vi "Merge Load Steps.vi"(9 "Load Steps  In 2":T1[](array[typedef]), 10 "Load Steps In":T1[](array[typedef])) -> (2 "Load Steps Out":T1[](array[typedef]))   [LabVIEW 2009]
uses:
  Load Step.ctl
  Widget/Target.ctl
  Data Access Objects/Metadata/LBCB Number.ctl
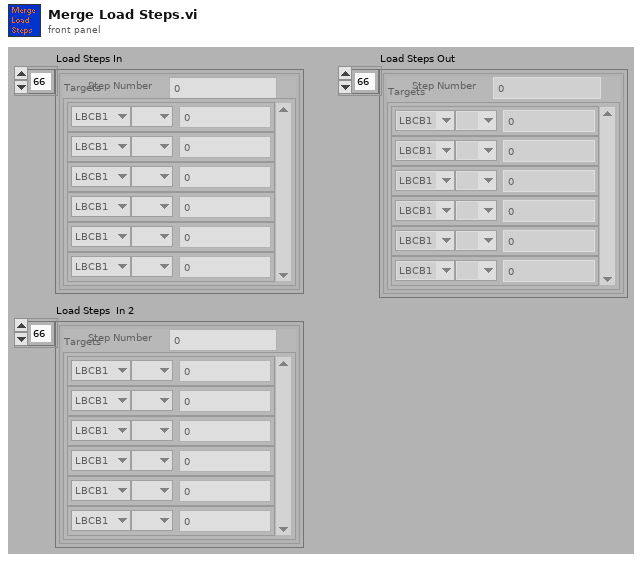
[diagram p1: front panel]
types:
  T1 = typedef "Load Step.ctl" = cluster{"Step Number":u32, "Targets":T2[]}
  T2 = typedef "Target.ctl" = cluster{"LBCB Number":T3, "DOF Vectors":enum16{" ", "Dx", "Dy", "Dz", "Rx", "Ry", "Rz", "Fx", "Fy", "Fz", "Mx", "My", "Mz"}, "Amount":dbl}
  T3 = typedef "LBCB Number.ctl" = enum16{"LBCB1", "LBCB2"}
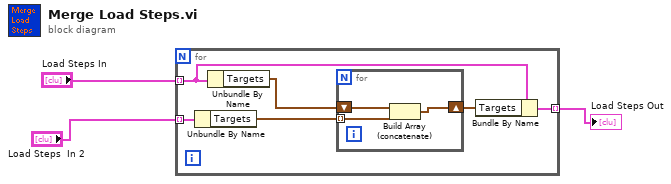
[diagram p0: block diagram]
diagram:
  n1 = for {
    tunnel: "Load Steps In" -> [w6] mode=indexing
    tunnel: "Load Steps  In 2" -> [w9] mode=indexing
    tunnel: [w4] -> w1 mode=indexing
    n2 = Unbundle By Name(w9) -> ("Targets"=w7:T2[])
    n3 = Unbundle By Name(w6) -> ("Targets"=w8:T2[])
    n4 = for {
      shift-right: [w11] -> w5
      shift-left: w8 -> [w12]
      tunnel: w7 -> [w10] mode=indexing
      n5 = Build Array (concatenate)(w12, w10) -> (w11:T2[])
    }
    n6 = Bundle By Name(cluster=w6, "Targets"=w5) -> (w4:T1)
  }
  "Load Steps Out" <- w1
